vi "Project List.vi"(4 "error in (no error)":errorcluster, 5 "LstBox Refnum":refnum<vi>, 6 "Project command":T1=enum."New project", 7 "User folder Path":path) -> (0 "error out":errorcluster, 3 "Project dates":timestamp[](array[timestamp]))   [LabVIEW 2015]
uses:
  Project commands.ctl
  AguaClara Library.lvlib
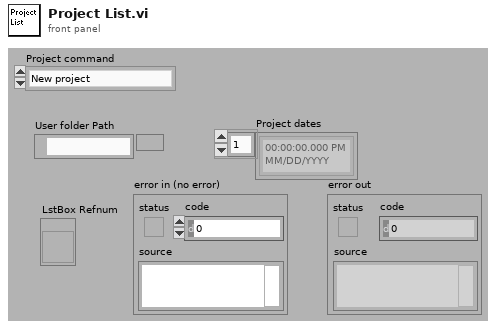
[diagram p1: front panel]
types:
  T1 = typedef "AguaClara Library.lvlib/Project commands.ctl" = enum16{"Load base file", "Load User", "Read paths", "Open Project", "New project", "Edit project", "Delete project", "Mail project", "save design", "open design"}
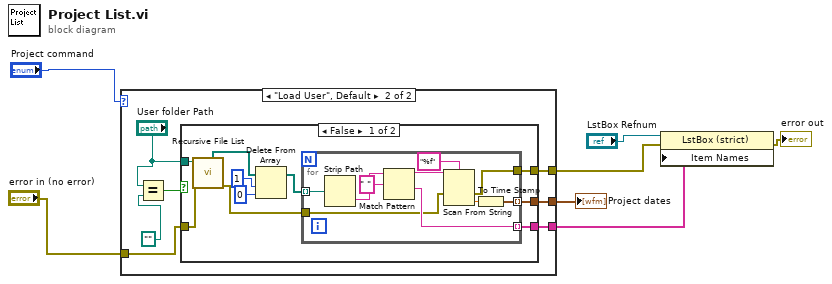
[diagram p0: block diagram]
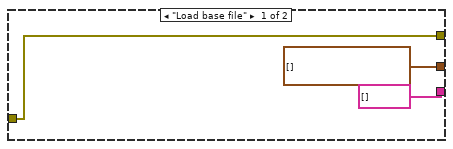
[diagram p2: hidden frame]
diagram:
  n1 = case shown="\"Load User\", Default" "Project command" {
    tunnel: [string[] [] w17] -> w5
    tunnel: [timestamp[] [] w16] -> w7
    tunnel: [w8 w12] -> w3
    tunnel: "error in (no error)" -> [w8 w11]
    frame "Load base file" {
    }
    frame "Load User", Default {
      n2 = Equal?(x="User folder Path", y=path "") -> (x = y?=w15:bool)
      n3 = case shown="False" w15 {
        tunnel: [w27 _] -> w17
        tunnel: [w26 _] -> w16
        tunnel: "User folder Path" -> [w25 _]
        tunnel: [w19 w38] -> w12
        tunnel: w11 -> [w18 w38]
        frame False {
          n4 = call <vilib>:"Recursive File List.vi"("error in (no error)"=w18, "Folder Path"=w25) -> ("error out"=w20:errorcluster, "All Folders"=w23:path[])  [unwired: 5 in, 3 out]
          n5 = Delete From Array(array=w23, length=1, index=0) -> (array with subset deleted=w24:path[])  [unwired: 1 out]
          n6 = for {
            tunnel: [w30] -> w26 mode=indexing
            tunnel: [w35] -> w27 mode=indexing
            tunnel: w24 -> [w33] mode=indexing
            tunnel: w20 -> [w29]
            tunnel: [w28] -> w19
            n7 = Strip Path(path=w33) -> (name=w32:string)  [unwired: 1 out]
            n8 = Match Pattern(string=w32, regular expression=" ") -> (before substring=w34:string, after substring=w35:string)  [unwired: 1 in, 2 out]
            n9 = Scan From String(format string="%f", input string=w34, error in=w29) -> (error out=w28:errorcluster, output 1=w31:dbl)  [unwired: 2 in, 2 out]
            n10 = To Time Stamp(1:w31) -> (0:w30:timestamp)
          }
        }
        frame True {
        }
      }
    }
  }
  "Project dates" <- w7
  n11 = property class="LstBox (strict)"(reference="LstBox Refnum", error in=w3, "Item Names"=w5) -> (error out=→"error out":errorcluster)  [unwired: 1 out]
